vi "Read Ocean optics configuration.vi"(8 "error in (no error)":errorcluster, 11 "Ocean Optics Driver in":refnum<class "Ocean Optics Driver.lvclass">) -> (0 "error out":errorcluster, 2 "Rubi spectra configuration":T1={"Integration time"=0.5, "Fit parameters"={"Peaks"=[{"Amplitude"=4000.0, "Center"=694.3, "Width"=0.4}, {"Amplitude"=2000.0, "Center"=692.8, "Width"=0.4}], "Function"=enum."Gauss", "Window width"=0.0}, "Fit"=FALSE, "Auto-update params"=FALSE, "Save spectra"=FALSE} {"Fit parameters"."Window width" format="%#_6gnm"; "Fit parameters"."Peaks"."Width" format="%#_gnm"; "Fit parameters"."Peaks"."Center" format="%#_gnm"; "Integration time" format="%#_6ps"}, 3 "Ocean Optics Driver out":refnum<class "Ocean Optics Driver.lvclass">)   [LabVIEW 2016, in "Ocean Optics Driver.lvclass"]
uses:
  Ocean Optics Driver.lvclass
  C:/github/NHMFL_Core/Libraries/Instruments/Instrument Driver/Instrument Driver.lvclass
  Ocean optics configuration.ctl
  Utilities/Fit/Multi-peak Parameters.ctl
  Utilities/Fit/Peak Parameters.ctl
  Instrument Driver/Read User configuration.vi
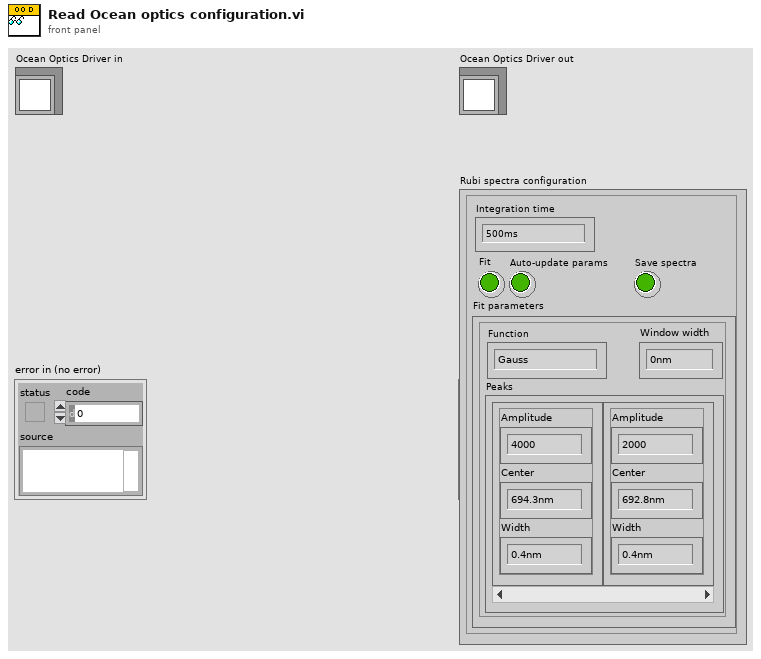
[diagram p1: front panel]
types:
  T1 = typedef "Ocean optics configuration.ctl" = cluster{"Integration time":dbl, "Fit parameters":T2, "Fit":bool, "Auto-update params":bool, "Save spectra":bool}
  T2 = typedef "Multi-peak Parameters.ctl" = cluster{"Peaks":T3[], "Function":enum16{"Gauss", "Lorentz"}, "Window width":dbl}
  T3 = typedef "Peak Parameters.ctl" = cluster{"Amplitude":dbl, "Center":dbl, "Width":dbl}
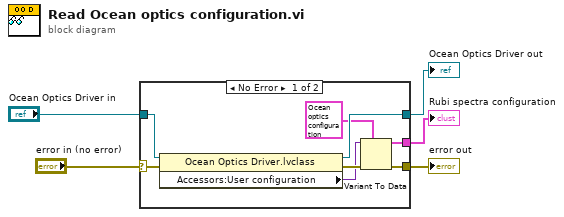
[diagram p0: block diagram]
diagram:
  n1 = case shown="No Error" "error in (no error)" {
    selector: "error in (no error)" -> [w13 w14]
    tunnel: [w9 w14] -> w4
    tunnel: [w10 w15] -> w2
    tunnel: "Ocean Optics Driver in" -> [w11 w15]
    tunnel: [w7 _] -> w1
    frame No Error {
      n2 = property class="Ocean Optics Driver.lvclass"(reference=w11, error in=w13) -> (reference out=w10:refnum<class "Ocean Optics Driver.lvclass">, error out=w12:errorcluster, "Accessors:User configuration"=w8:variant)
      n3 = Variant To Data(error in=w12, type=T1 {"Integration time"=0.5, "Fit parameters"={"Peaks"=[{"Amplitude"=4000.0, "Center"=694.3, "Width"=0.4}, {"Amplitude"=2000.0, "Center"=692.8, "Width"=0.4}], "Function"=enum."Gauss", "Window width"=0.0}, "Fit"=FALSE, "Auto-update params"=FALSE, "Save spectra"=FALSE} ("Rubi spectra configuration"), Variant=w8) -> (data=w7:T1, error out=w9:errorcluster)
    }
    frame Error {
    }
  }
  "error out" <- w4
  "Ocean Optics Driver out" <- w2
  "Rubi spectra configuration" <- w1
